vi "Set Wavelength.vi"(7 "Simulation":T2, 8 "error in":errorcluster, 9 "String":string, 10 "Args":string[](array[string]), 11 "Ophir Pulsar in":refnum<class "Ophir Juno.lvclass">) -> (0 "error out":errorcluster, 2 "new commands":string, 3 "Ophir Pulsar out":refnum<class "Ophir Juno.lvclass">)   [LabVIEW 2020, in "Ophir Juno.lvclass"]
uses:
  Ophir Juno.lvclass
  shared/OnOffTypeDef.ctl
  Controls/Wavelength.ctl
  Ophir Juno.lvclass/Ophir Juno.ctl
  shared/CompressAndUpdate(Poly)/CompressAndUpdate(Enum).vi
panel:
  in  "Wavelength(nm)":T1
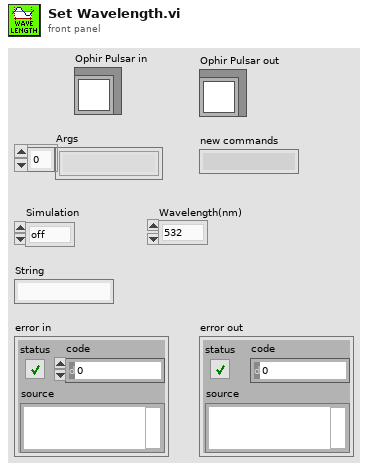
[diagram p1: front panel]
types:
  T1 = typedef "Ophir Juno.lvclass/Wavelength.ctl" = enum16{"532", "800"}
  T2 = typedef "OnOffTypeDef.ctl" = enum16{"off", "on"}
  T3 = cluster{"Channel0":T1, "Channel1":T1, "Channel2":T1, "Channel3":T1}
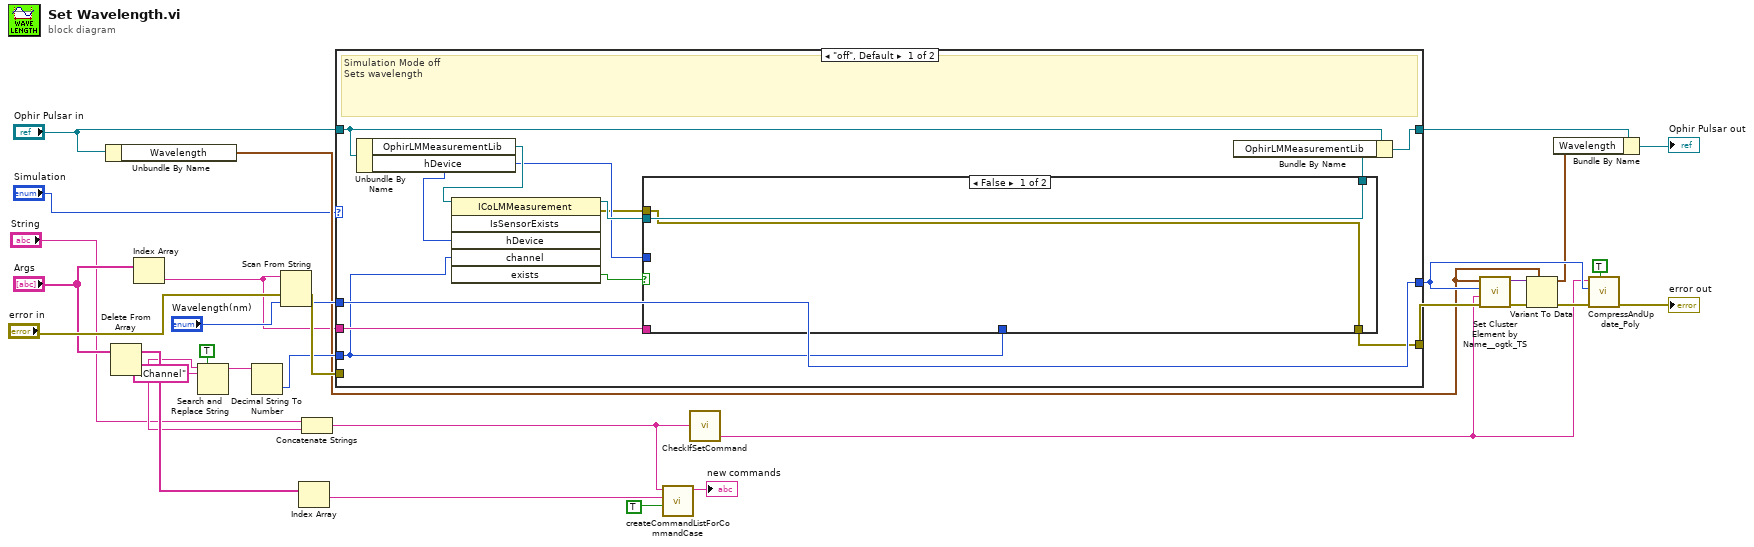
[diagram p0: block diagram]
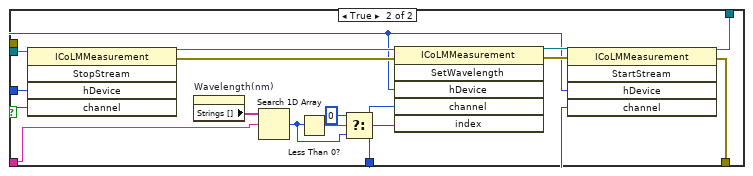
[diagram p2: hidden frame]
diagram:
  n1 = Unbundle By Name("Ophir Pulsar in") -> ("Wavelength"=w14:T3)
  n2 = Delete From Array(array="Args") -> (deleted portion=w12:string, array with subset deleted=w18:string[])  [unwired: 2 in]
  n3 = Index Array(array="Args") -> (element=w1:string)  [unwired: 1 in]
  n4 = Search and Replace String(replace all?=TRUE ("replace all? (F)"), input string=w12, search string=".Channel") -> (result string=w16:string)  [unwired: 5 in, 3 out]
  n5 = Decimal String To Number(string=w16) -> (number=w30:i32)  [unwired: 2 in, 1 out]
  n6 = Scan From String(input string=w1, error in="error in", default 1="Wavelength(nm)") -> (error out=w31:errorcluster, output 1=w24:T1)  [unwired: 2 in, 2 out]
  n7 = Index Array(array=w18) -> (element=w19:string)  [unwired: 1 in]
  n8 = Concatenate Strings("String", w12) -> (w17:string)
  n9 = case shown="\"off\", Default" "Simulation" {
    tunnel: w24 -> [w41 w63]
    tunnel: [w41 w63] -> w26
    tunnel: w31 -> [_ w62]
    tunnel: [w40 w62] -> w27
    tunnel: "Ophir Pulsar in" -> [w43 w61]
    tunnel: [w42 w61] -> w21
    tunnel: w30 -> [w34 _]
    tunnel: w1 -> [w38 _]
    frame "off", Default {
      # "Simulation Mode off\nSets wavelength"
      n10 = Unbundle By Name(w43) -> ("OphirLMMeasurementLib"=w37:refnum<k7>, "hDevice"=w35:i32)
      n11 = invoke class="ICoLMMeasurement" method="IsSensorExists"(reference=w37, "hDevice"=w35, "channel"=w34) -> (reference out=w36:refnum<k7>, error out=w32:errorcluster, "exists"=w33:bool)  [unwired: 3 in, 3 out]
      n12 = case shown="False" w33 {
        tunnel: [w44 w56] -> w40
        tunnel: [w45 w55] -> w39
        tunnel: w38 -> [_ w49]
        tunnel: w36 -> [w45 w48]
        tunnel: w35 -> [_ w47]
        tunnel: w34 -> [_ w46]
        tunnel: w32 -> [w44 _]
        frame False {
        }
        frame True {
          n13 = invoke class="ICoLMMeasurement" method="StopStream"(reference=w48, "hDevice"=w47, "channel"=w46) -> (reference out=w59:refnum<k7>, error out=w60:errorcluster)  [unwired: 2 in, 3 out]
          n14 = property on="Wavelength(nm)" class="Enum (strict)"() -> ("Strings []"=w54:string[])  [unwired: 2 in, 2 out]
          n15 = Search 1D Array(1D array=w54, element=w49) -> (index of element=w51:i32)  [unwired: 1 in]
          n16 = Less Than 0?(x=w51) -> (x < 0?=w53:bool)
          n17 = Select(t=0, s=w53, f=w51) -> (s? t:f=w50:i32)
          n18 = invoke class="ICoLMMeasurement" method="SetWavelength"(reference=w59, error in=w60, "hDevice"=w47, "channel"=w46, "index"=w50) -> (reference out=w58:refnum<k7>, error out=w57:errorcluster)  [unwired: 1 in, 4 out]
          n19 = invoke class="ICoLMMeasurement" method="StartStream"(reference=w58, error in=w57, "hDevice"=w47, "channel"=w46) -> (reference out=w55:refnum<k7>, error out=w56:errorcluster)  [unwired: 1 in, 3 out]
        }
      }
      n20 = Bundle By Name(cluster=w43, "OphirLMMeasurementLib"=w39) -> (w42:refnum<class "Ophir Juno.lvclass">)
    }
    frame "on" {
      # "Simulation Mode on"
    }
  }
  n21 = call "createCommandListForCommandCase.vi"("immediate Check (only once)"=TRUE, "setvalue"=w19, "command"=w17) -> ("new commands"=→"new commands":string)  [unwired: 8 in]
  n22 = call "CheckIfSetCommand.vi"("Command"=w17) -> ("variable"=w11:string)  [unwired: 2 out]
  n23 = call "Set Cluster Element by Name__ogtk_TS.vi"("error in (no error)"=w27, "Element Name (\"\": New Element Data Name)"=w11, "New Element Value"=w26, "Cluster"=w14) -> ("error out"=w28:errorcluster, "VCluster out"=w15:variant)  [unwired: 5 in, 1 out]
  n24 = Variant To Data(error in=w28, type=w14, Variant=w15) -> (data=w13:T3, error out=w29:errorcluster)
  n25 = Bundle By Name(cluster=w21, "Wavelength"=w13) -> (→"Ophir Pulsar out":refnum<class "Ophir Juno.lvclass">)
  n26 = call-poly "CompressAndUpdate_Poly.vi"("force CVT update (false)"=TRUE, "error in"=w29, "enum variant"=w26, "command or variable name"=w11) -> ("error out"=→"error out":errorcluster)  [unwired: 7 in]
